vi "Set DPD LUT Name.vi"(8 "error in (no error)":errorcluster, 10 "DPD LUT Name":string, 11 "Test Group In":refnum<data-value>) -> (0 "error out":errorcluster, 3 "Test Group Out":refnum<data-value>)   [LabVIEW 2016, in "Test Group Manager.lvlib" / "Test Group.lvclass"]
uses:
  Test Group.lvclass
  Test Group.lvclass/Test Group.ctl
  Read Test Group Data.vi
  Write Test Group Data.vi
  Write DPD Initialized.vi
  Read DPD Initialized.vi
  <vilib>/Utility/error.llb/Error Cluster From Error Code.vi
  <vilib>/ErrorRing/Error Ring.xnode
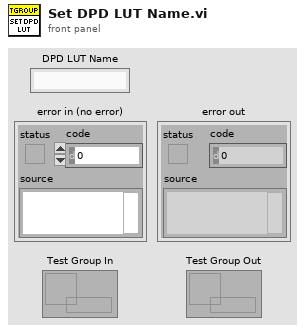
[diagram p1: front panel]
types:
  T1 = cluster{"DPD LUT Name":string, "Input Power":string}
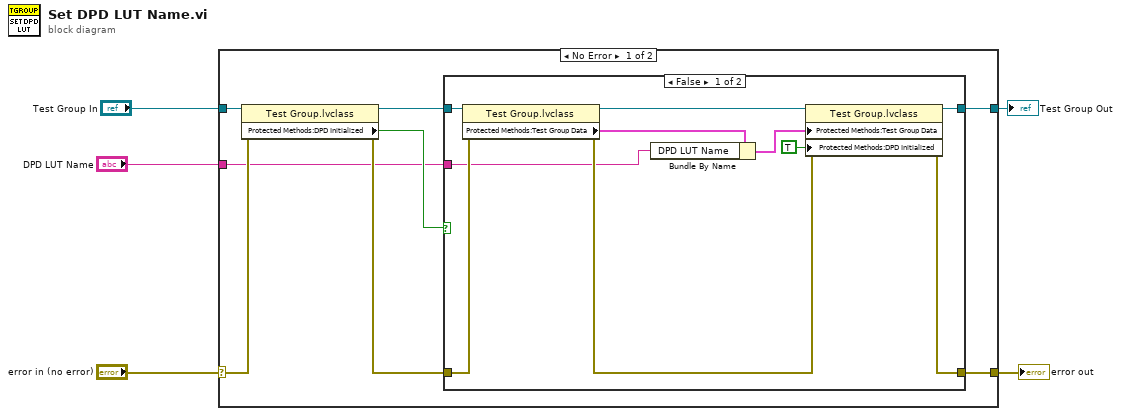
[diagram p0: block diagram]
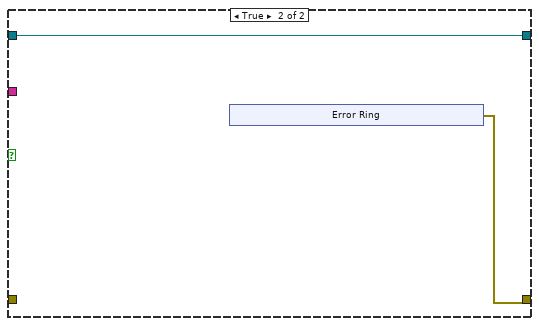
[diagram p2: hidden frame]
diagram:
  n1 = case shown="No Error" "error in (no error)" {
    selector: "error in (no error)" -> [w13 w32]
    tunnel: [w11 w32] -> w4
    tunnel: [w8 w31] -> w1
    tunnel: "Test Group In" -> [w12 w31]
    tunnel: "DPD LUT Name" -> [w6 _]
    frame No Error {
      n2 = property class="Test Group.lvclass"(reference=w12, error in=w13) -> (reference out=w7:refnum<data-value>, error out=w10:errorcluster, "Protected Methods:DPD Initialized"=w9:bool)
      n3 = case shown="False" w9 {
        tunnel: [w22 w25] -> w11
        tunnel: w10 -> [w23 _]
        tunnel: [w21 w24] -> w8
        tunnel: w7 -> [w19 w24]
        tunnel: w6 -> [w15 _]
        frame False {
          n4 = property class="Test Group.lvclass"(reference=w19, error in=w23) -> (reference out=w18:refnum<data-value>, error out=w20:errorcluster, "Protected Methods:Test Group Data"=w17:T1)
          n5 = Bundle By Name(cluster=w17, "DPD LUT Name"=w15) -> (w16:T1)
          n6 = property class="Test Group.lvclass"(reference=w18, error in=w20, "Protected Methods:Test Group Data"=w16, "Protected Methods:DPD Initialized"=TRUE ("DPD Initialized")) -> (reference out=w21:refnum<data-value>, error out=w22:errorcluster)
        }
        frame True {
          n7 = xnode "Error Ring"() -> ("error out"=w25:errorcluster)
        }
      }
    }
    frame Error {
    }
  }
  "error out" <- w4
  "Test Group Out" <- w1
